vi "MsgQue.vi"() -> ()   [LabVIEW 2019, in "MsgShowAndLog.lvlib"]
uses:
  MsgShowAndLog.lvlib
  Ctrl/MsgDataInput.ctl
  Ctrl/MsgPageSelect.ctl
  Ctrl/LogType.ctl
panel:
  out "MsgQue":refnum<queue>
  in  "Btn_Exit":refnum<vi>
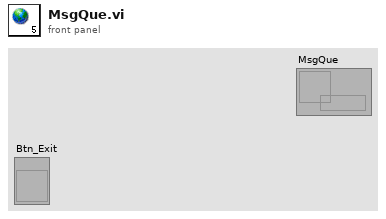
[diagram p1: front panel]
diagram:
